vi "Wait.vi"(0 "object in":refnum<class "Application.lvclass">, 2 "Time Target (s)":dbl=1.0, 5 "error in (no error)":errorcluster) -> (14 "object out":refnum<class "Application.lvclass">, 19 "error out":errorcluster)   [LabVIEW 2019, in "Application.lvclass"]
uses:
  Application.lvclass
  Application.lvclass/Application.ctl
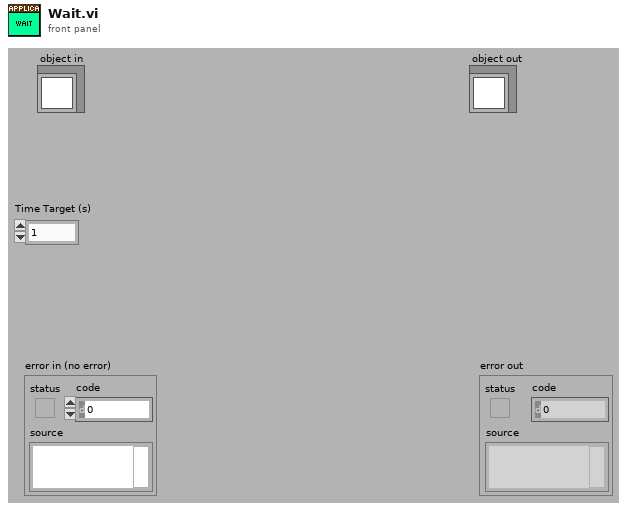
[diagram p1: front panel]
types:
  T1 = cluster{"Message":string, "Message Data":variant}
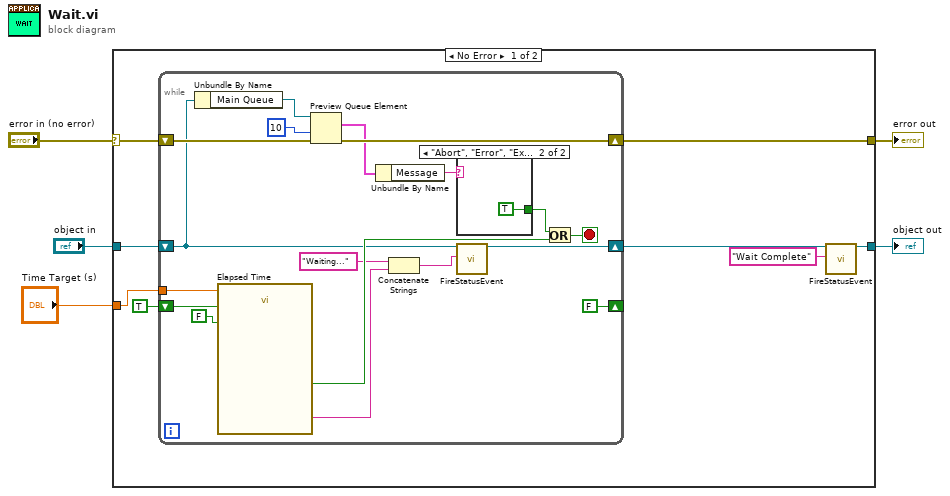
[diagram p0: block diagram]
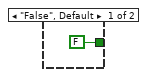
[diagram p2: hidden frame]
diagram:
  n1 = case shown="No Error" "error in (no error)" {
    selector: "error in (no error)" -> [w12 w35]
    tunnel: [w11 w35] -> w4
    tunnel: [w7 w34] -> w2
    tunnel: "object in" -> [w13 w34]
    tunnel: "Time Target (s)" -> [w10 _]
    frame No Error {
      n2 = while {
        tunnel: w10 -> [w25]
        shift-right: [w28] -> w11
        shift-left: w12 -> [w29]
        shift-right: [w17] -> w8
        shift-left: w13 -> [w18]
        shift-right: [FALSE] -> _
        shift-left: TRUE -> [w20]
        stop <- w23 stop-if-true
        n3 = Unbundle By Name(w18) -> ("Main Queue"=w31:refnum<queue>)
        n4 = call "Elapsed Time"("Time Target (s)"=w25, "Reset"=w20, "Auto Reset"=FALSE) -> ("Time has Elapsed"=w22:bool, "Elapsed Time Text"=w15:string)  [unwired: 9 in, 6 out]
        n5 = Preview Queue Element(queue=w31, timeout in ms (-1)=10, error in (no error)=w29) -> (element=w27:T1, error out=w28:errorcluster)  [unwired: 2 out]
        n6 = Unbundle By Name(w27) -> ("Message"=w26:string)
        n7 = Concatenate Strings("Waiting..." ("string"), w15) -> (w14:string)
        n8 = case shown="\"Abort\", \"Error\", \"Exit\"" w26 {
          tunnel: [FALSE TRUE] -> w24
          frame "False", Default {
          }
          frame "Abort", "Error", "Exit" {
          }
        }
        n9 = call-dynamic "FireStatusEvent.vi"("object in"=w18, "Status"=w14) -> ("object out"=w17:refnum<class "Application.lvclass">)  [unwired: 16 in, 1 out]
        n10 = Or(x=w24, y=w22) -> (x .or. y?=w23:bool)
      }
      n11 = call-dynamic "FireStatusEvent.vi"("object in"=w8, "Status"="Wait Complete") -> ("object out"=w7:refnum<class "Application.lvclass">)  [unwired: 16 in, 1 out]
    }
    frame Error {
    }
  }
  "error out" <- w4
  "object out" <- w2
